vi "Plot StringToFormatCode.vi"(11 "Start String":string) -> (0 "Error":bool, 1 "FormatCode":T1, 2 "Delim":string, 3 "Remaining String":string)   [LabVIEW 2020, in "3D Plot.lvclass"]
uses:
  3D Plot.lvclass
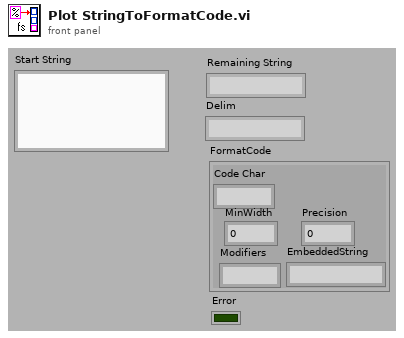
[diagram p1: front panel]
types:
  T1 = cluster{"Code Char":string, "Precision":i32, "MinWidth":u16, "EmbeddedString":string, "Modifiers":string}
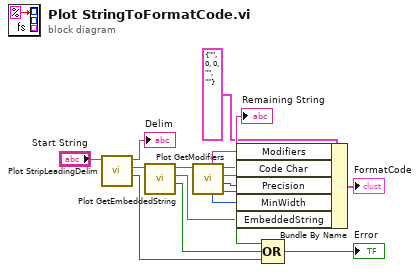
[diagram p0: block diagram]
diagram:
  n1 = call "Plot StripLeadingDelim.vi"("Start String"="Start String") -> ("Error"=w6:bool, "Remaining String"=w13:string, "Delim"=→"Delim":string)  [unwired: 8 out]
  n2 = call "Plot GetEmbeddedString.vi"("Start String"=w13) -> ("Error"=w2:bool, "EmbeddedString"=w3:string, "Remaining String"=w12:string)  [unwired: 8 out]
  n3 = call "Plot GetModifiers.vi"("Start String"=w12) -> ("Error"=w5:bool, "Precision"=w10:i32, "Code Character"=w9:string, "Remaining String"=→"Remaining String":string, "Min Width"=w11:u16, "Modifiers"=w8:string)  [unwired: 5 out]
  n4 = Bundle By Name(cluster=T1 {"Code Char"="", "Precision"=0, "MinWidth"=0, "EmbeddedString"="", "Modifiers"=""} ("FormatCode"), "Modifiers"=w8, "Code Char"=w9, "Precision"=w10, "MinWidth"=w11, "EmbeddedString"=w3) -> (→"FormatCode":T1)
  n5 = Compound Arithmetic op=OR(w5, w2, w6) -> (→"Error":bool)
